vi "Obtain Request Events.vi"(8 "error in":errorcluster, 10 "Create New? (F)":bool) -> (0 "error out":errorcluster, 2 "UIs Handler Request Events":T1)   [LabVIEW 2024, in "UIs Handler.lvlib"]
doc: "This VI Obtains/Creates the Requests events that will be used for other modules to communicate with the module that owns this VI. These Requests events will be accessed only via Public API methods for this module.\n\n<b>NOTE</b>: The contents of this VI are automatically generated and modified by the <b>Tools > DQMH Consortium > DQMH</b> utilities. Consider using those utilities instead of making your own modifications to this VI.\n_____\nBased on DQMH Dev Tools: Project Template 7.1.0.1490."
uses:
  UIs Handler.lvlib
  Request Events--cluster.ctl
  Stop Argument--cluster.ctl
  Show Panel Argument--cluster.ctl
  Hide Panel Argument--cluster.ctl
  Get Module Execution Status Argument--cluster.ctl
  Show Diagram Argument--cluster.ctl
  Insert UI into subpanel Argument--cluster.ctl
  UIs/Select UI.ctl
  Start Counter Argument--cluster.ctl
  Reset Counter Argument--cluster.ctl
  Save Counter Argument--cluster.ctl
  Dashboard HLwakeup Argument--cluster.ctl
  Start Dashboard Monitoring Argument--cluster.ctl
panel:
  # "NOTE: The contents of this VI are automatically generated and modified by the Tools > DQMH Consortium > DQMH utilities. Consider using those utilities instead of making your own modifications to this VI."
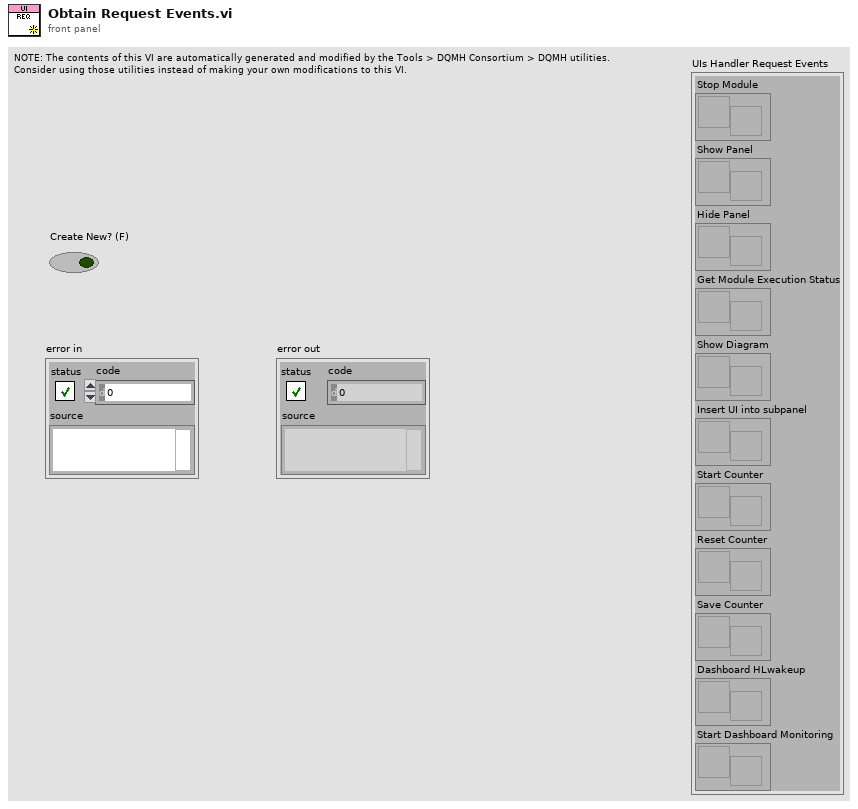
[diagram p1: front panel]
types:
  T1 = typedef "UIs Handler.lvlib/Request Events--cluster.ctl" = cluster{"Stop Module":refnum<user-event>, "Show Panel":refnum<user-event>, "Hide Panel":refnum<user-event>, "Get Module Execution Status":refnum<user-event>, "Show Diagram":refnum<user-event>, "Insert UI into subpanel":refnum<user-event>, "Start Counter":refnum<user-event>, "Reset Counter":refnum<user-event>, "Save Counter":refnum<user-event>, "Dashboard HLwakeup":refnum<user-event>, "Start Dashboard Monitoring":refnum<user-event>}
  T2 = typedef "UIs Handler.lvlib/Start Dashboard Monitoring Argument--cluster.ctl" = cluster{"Boolean":bool}
  T3 = typedef "UIs Handler.lvlib/Dashboard HLwakeup Argument--cluster.ctl" = cluster{"Boolean":bool}
  T4 = typedef "UIs Handler.lvlib/Save Counter Argument--cluster.ctl" = cluster{"Boolean":bool}
  T5 = typedef "UIs Handler.lvlib/Reset Counter Argument--cluster.ctl" = cluster{"Boolean":bool}
  T6 = typedef "UIs Handler.lvlib/Start Counter Argument--cluster.ctl" = cluster{"Boolean":bool}
  T7 = typedef "UIs Handler.lvlib/Insert UI into subpanel Argument--cluster.ctl" = cluster{"Subpanel":refnum<vi>, "Select UI":T8}
  T8 = typedef "UIs Handler.lvlib/Select UI.ctl" = enum16{"Dashboard", "Meta Tabs"}
  T9 = typedef "UIs Handler.lvlib/Hide Panel Argument--cluster.ctl" = cluster{"Hide Panel?":bool}
  T10 = typedef "UIs Handler.lvlib/Show Panel Argument--cluster.ctl" = cluster{"Show Panel?":bool}
  T11 = typedef "UIs Handler.lvlib/Show Diagram Argument--cluster.ctl" = cluster{"Debug?":bool}
  T12 = typedef "UIs Handler.lvlib/Get Module Execution Status Argument--cluster.ctl" = cluster{"Running?":bool}
  T13 = typedef "UIs Handler.lvlib/Stop Argument--cluster.ctl" = cluster{"Origin":string, "Exit via Stop Module Req?":bool, "Wait for Module to stop?":bool}
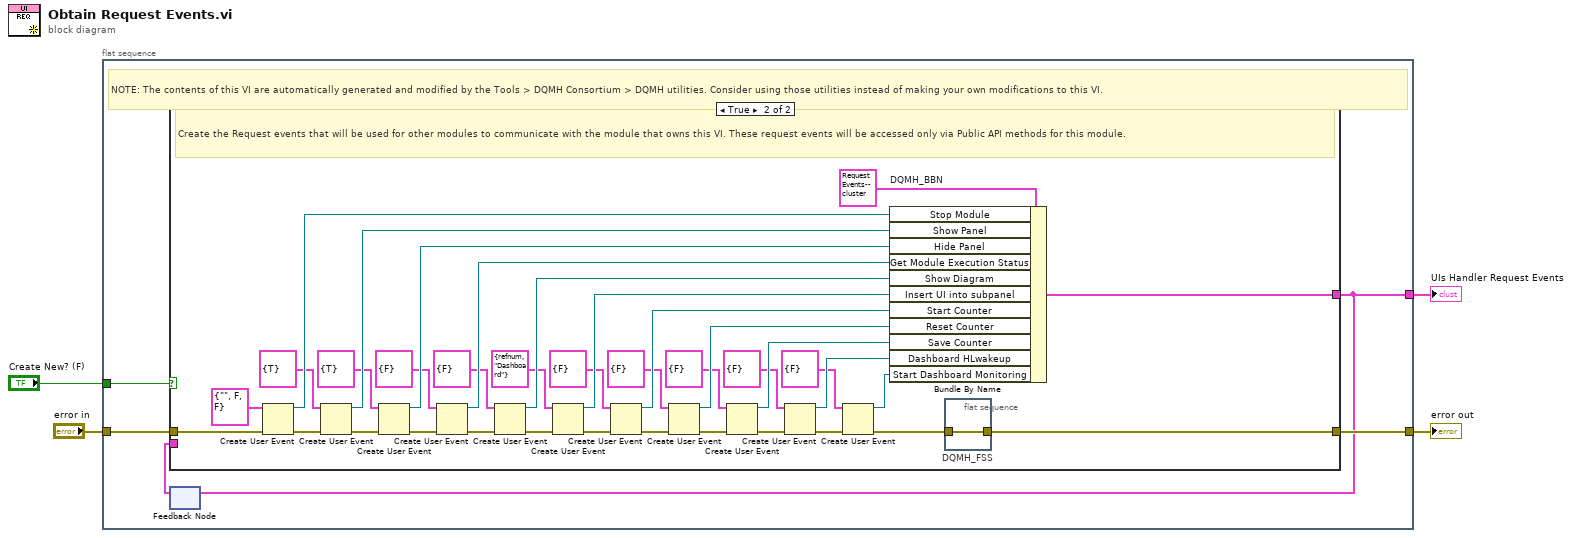
[diagram p0: block diagram]
diagram:
  n1 = flat-sequence {
    tunnel: [w9] -> w4
    tunnel: "error in" -> [w8]
    tunnel: [w6] -> w2
    tunnel: "Create New? (F)" -> [w5]
    frame #0 {
      # "NOTE: The contents of this VI are automatically generated and modified by the Tools > DQMH Consortium > DQMH utilities. Consider using those utilities instead of making your own modifications to this VI."
      n2 = feedback #1() -> (w7:T1)  [unwired: 1 in]
      n3 = case shown="True" w5 {
        tunnel: [w10 w38] -> w9
        tunnel: w8 -> [w10 w48]
        tunnel: [w11 w45] -> w6
        tunnel: w7 -> [w11 _]
        frame False {
          # "Obtain the Request events that were created in a previous call to this VI."
        }
        frame True {
          # "Create the Request events that will be used for other modules to communicate with the module that owns this VI. These request events will be accessed only via Public API methods for this module."
          n4 = Create User Event(user event datatype=T13 {"Origin"="", "Exit via Stop Module Req?"=FALSE, "Wait for Module to stop?"=FALSE} ("Stop Argument"), error in=w48) -> (user event=w46:refnum<user-event>, error out=w43:errorcluster)
          n5 = Create User Event(user event datatype=T10 {"Show Panel?"=TRUE} ("Show Panel Argument"), error in=w43) -> (user event=w42:refnum<user-event>, error out=w41:errorcluster)
          n6 = Create User Event(user event datatype=T9 {"Hide Panel?"=TRUE} ("Hide Panel Argument"), error in=w41) -> (user event=w40:refnum<user-event>, error out=w39:errorcluster)
          n7 = Create User Event(user event datatype=T12 {"Running?"=FALSE} ("Get Module Execution Status Argument"), error in=w39) -> (user event=w36:refnum<user-event>, error out=w37:errorcluster)
          n8 = Create User Event(user event datatype=T11 {"Debug?"=FALSE} ("Show Diagram Argument"), error in=w37) -> (user event=w33:refnum<user-event>, error out=w34:errorcluster)
          n9 = Create User Event(user event datatype=T7 {"Subpanel"=refnum, "Select UI"=enum."Dashboard"} ("Insert UI into subpanel Argument"), error in=w34) -> (user event=w28:refnum<user-event>, error out=w29:errorcluster)
          n10 = Create User Event(user event datatype=T6 {"Boolean"=FALSE} ("Start Counter Argument"), error in=w29) -> (user event=w25:refnum<user-event>, error out=w26:errorcluster)
          n11 = Create User Event(user event datatype=T5 {"Boolean"=FALSE} ("Reset Counter Argument"), error in=w26) -> (user event=w22:refnum<user-event>, error out=w23:errorcluster)
          n12 = Create User Event(user event datatype=T4 {"Boolean"=FALSE} ("Save Counter Argument"), error in=w23) -> (user event=w19:refnum<user-event>, error out=w20:errorcluster)
          n13 = Create User Event(user event datatype=T3 {"Boolean"=FALSE} ("Dashboard HLwakeup Argument"), error in=w20) -> (user event=w16:refnum<user-event>, error out=w17:errorcluster)
          n14 = Create User Event(user event datatype=T2 {"Boolean"=FALSE} ("Start Dashboard Monitoring Argument"), error in=w17) -> (user event=w13:refnum<user-event>, error out=w14:errorcluster)
          n15 = Bundle By Name "DQMH_BBN"(cluster=T1 {"Stop Module"=refnum, "Show Panel"=refnum, "Hide Panel"=refnum, "Get Module Execution Status"=refnum, "Show Diagram"=refnum, "Insert UI into subpanel"=refnum, "Start Counter"=refnum, "Reset Counter"=refnum, "Save Counter"=refnum, "Dashboard HLwakeup"=refnum, "Start Dashboard Monitoring"=refnum} ("output cluster"), "Stop Module"=w46, "Show Panel"=w42, "Hide Panel"=w40, "Get Module Execution Status"=w36, "Show Diagram"=w33, "Insert UI into subpanel"=w28, "Start Counter"=w25, "Reset Counter"=w22, "Save Counter"=w19, "Dashboard HLwakeup"=w16, "Start Dashboard Monitoring"=w13) -> (w45:T1)
          n16 = flat-sequence "DQMH_FSS" {
            tunnel: w14 -> [w49]
            tunnel: [w49] -> w38
            frame #0 {
            }
          }
        }
      }
      n17 = feedback-in #1(w6) -> ()
    }
  }
  "UIs Handler Request Events" <- w2
  "error out" <- w4
